vi "structure full adder.vi"(2 "c":bool, 3 "B":bool, 4 "a":bool) -> (0 "carry":bool, 1 "sum":bool)   [LabVIEW 2017]
panel:
  in  "Boolean":bool
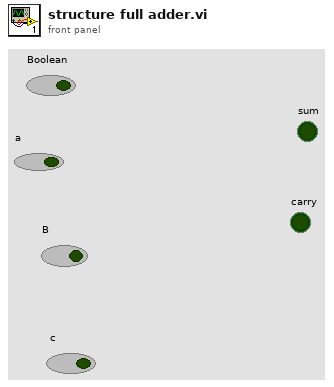
[diagram p1: front panel]
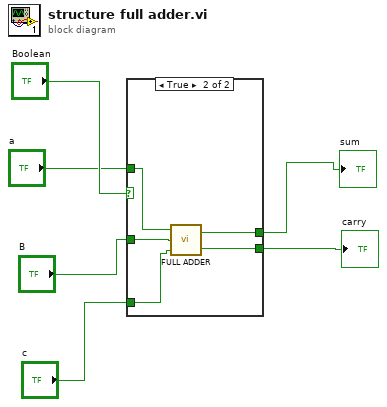
[diagram p0: block diagram]
diagram:
  n1 = case shown="True" "Boolean" {
    tunnel: "a" -> [_ w11]
    tunnel: "B" -> [_ w10]
    tunnel: "c" -> [_ w9]
    tunnel: [_ w8] -> w2
    tunnel: [_ w7] -> w1
    frame False {
    }
    frame True {
      n2 = call "FULL ADDER.vi"("C"=w9, "B"=w10, "A"=w11) -> ("CARRY"=w7:bool, "SUM"=w8:bool)
    }
  }
  "sum" <- w2
  "carry" <- w1
